vi "CalculateVSTLevels.vi"(8 "error in":errorcluster, 9 "Waveform":T2={"Waveform Name"="Wfm", "Waveform"={"x0"=0.0, "dx"=0.0, "y"=[]}, "Signal Bandwidth (Hz)"=0.0, "PAPR (dB)"=0.0, "Burst Length (s)"=0.0, "Sample Rate"=0.0, "Burst Start Locations"=[], "Burst Stop Locations"=[], "Idle Duration Present?"=FALSE, "Runtime Scaling"=0.0} {"Runtime Scaling" format="%#_6p"; "Sample Rate" format="%#_6p"; "Burst Length (s)" format="%#_6p"; "PAPR (dB)" format="%.2f"; "Signal Bandwidth (Hz)" format="%#_6p"; "Waveform"."y" format="%.2f"; "Waveform"."dx" format="%^.2e"; "Waveform"."x0" format="%^.2e"}, 10 "DUT Configuration":T3 {"DUT Gain Accuracy (dB)" format="%.2g"; "DUT Estimated Gain (dBm)" format="%.2g"; "DUT Desired Output Power (dBm)" format="%.2g"}, 11 "servoSessionIn":u32) -> (0 "error out":errorcluster, 2 "CalculatedVSTLevels":T1, 3 "servoSessionOut":u32)   [LabVIEW 2016, in "Power Servo.lvlib"]
uses:
  Power Servo.lvlib
  Type Definitions/Dut Configuration.ctl
  SG/Typedefs/Waveform.ctl
  Type Definitions/CalculatedVSTLevels.ctl
  <userlib>/_NI Power Servoing IP/HostRdl/NI Power Servoing IP New (Host).lvlib
  SG/SG.lvlib
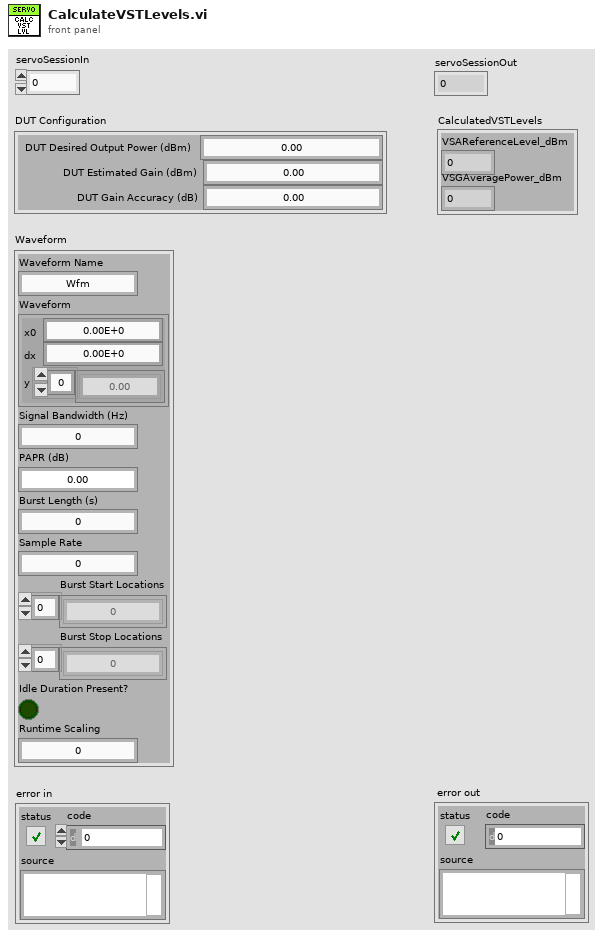
[diagram p1: front panel]
types:
  T1 = typedef "CalculatedVSTLevels.ctl" = cluster{"VSAReferenceLevel_dBm":dbl, "VSGAveragePower_dBm":dbl}
  T2 = typedef "SG.lvlib/Waveform.ctl" = cluster{"Waveform Name":string, "Waveform":cluster{"x0":dbl, "dx":dbl, "y":csg[]}, "Signal Bandwidth (Hz)":dbl, "PAPR (dB)":dbl, "Burst Length (s)":dbl, "Sample Rate":dbl, "Burst Start Locations":i32[], "Burst Stop Locations":i32[], "Idle Duration Present?":bool, "Runtime Scaling":dbl}
  T3 = typedef "Power Servo.lvlib/Dut Configuration.ctl" = cluster{"DUT Desired Output Power (dBm)":dbl, "DUT Estimated Gain (dBm)":dbl, "DUT Gain Accuracy (dB)":dbl}
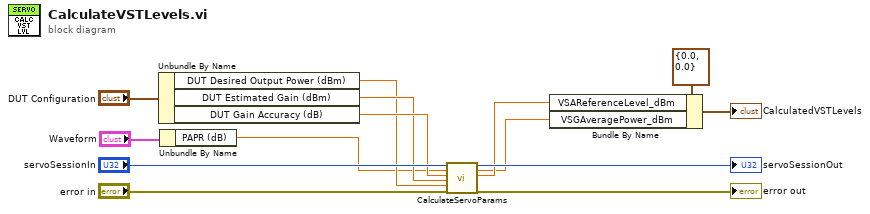
[diagram p0: block diagram]
diagram:
  n1 = Unbundle By Name("DUT Configuration") -> ("DUT Desired Output Power (dBm)"=w8:dbl, "DUT Estimated Gain (dBm)"=w9:dbl, "DUT Gain Accuracy (dB)"=w10:dbl)
  n2 = Unbundle By Name("Waveform") -> ("PAPR (dB)"=w1:dbl)
  n3 = call <userlib>:"CalculateServoParams.vi"("SessionHandleIn"="servoSessionIn", "MeasurementHeadroomDB"=w1, "GainAccuracyDB"=w10, "EstimatedPAGainDB"=w9, "DesiredPAOutputPowerDBm"=w8, "error in"="error in") -> ("SessionHandleOut"=→"servoSessionOut":u32, "VSGAveragePowerDBm"=w3:dbl, "ReferenceLevelDBm"=w4:dbl, "error out"=→"error out":errorcluster)  [unwired: 10 in]
  n4 = Bundle By Name(cluster=T1 {"VSAReferenceLevel_dBm"=0.0, "VSGAveragePower_dBm"=0.0} ("CalculatedVSTLevels"), "VSAReferenceLevel_dBm"=w4, "VSGAveragePower_dBm"=w3) -> (→"CalculatedVSTLevels":T1)
